vi "Register Discovered Object Instance (incoming).vi"(10 "discoverObjInstance":T1, 11 "hlaMap in":T2) -> (3 "hlaMap out":T2)   [LabVIEW 2019, in "HLA Custom Device Engine.lvlib"]
uses:
  HLA Custom Device Engine.lvlib
  map_object_instance_value.ctl
  _Debug/VsDebugLibrary.lvlib
  map_attr_param_data.ctl
  map_interaction_value.ctl
  map_interaction.ctl
  map_object_value.ctl
  map_object_key.ctl
  map_object.ctl
  map_object_instance.ctl
  map_object_vs_instance.ctl
  RThlaMapHelpers.ctl
  discoverObjectInstance_type.ctl
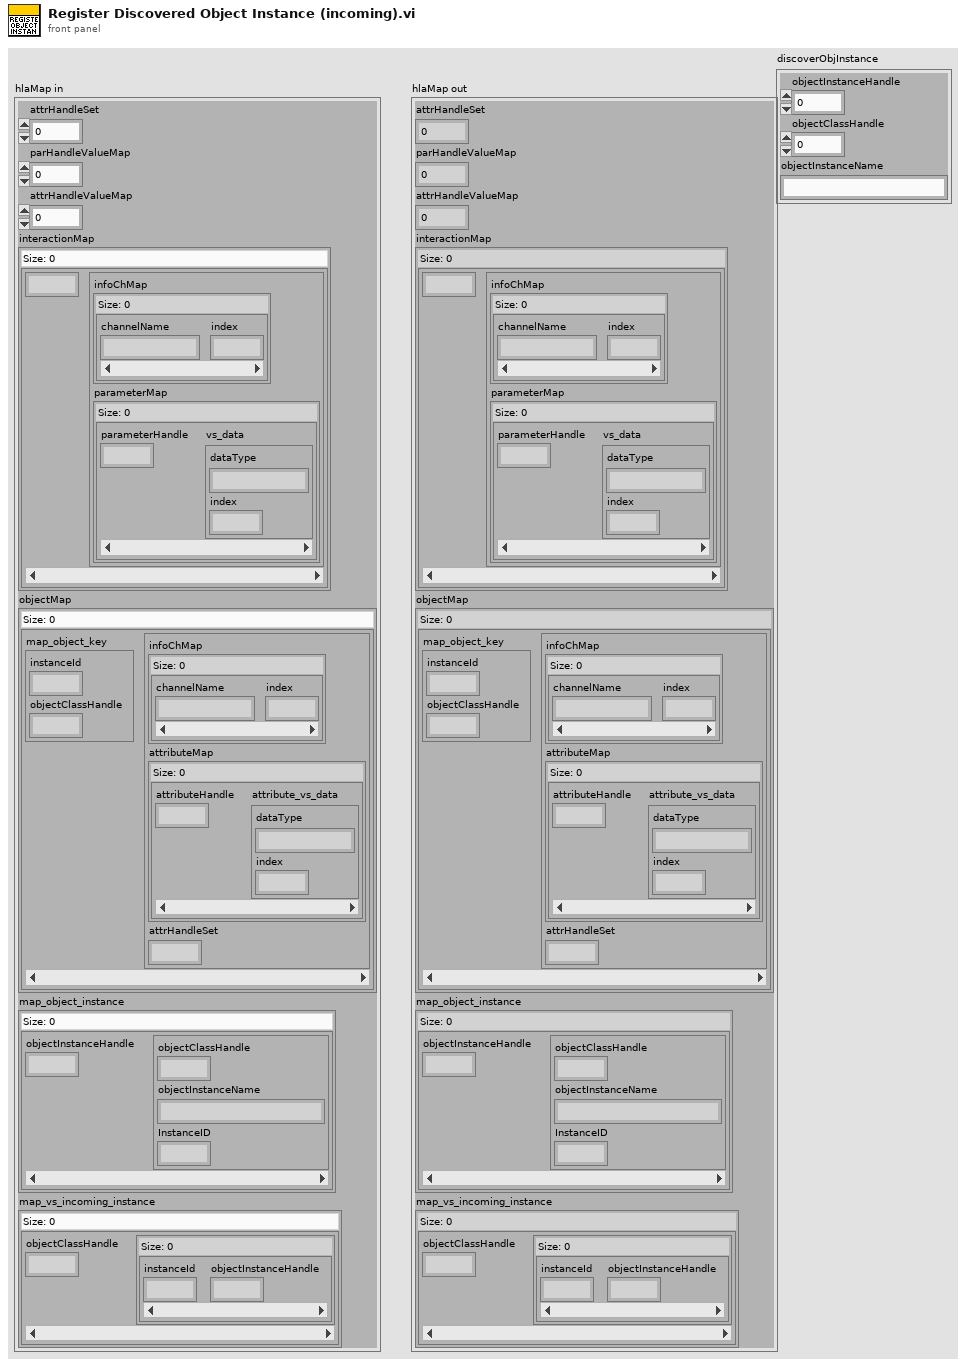
[diagram p1: front panel]
types:
  T1 = typedef "HLA Custom Device Engine.lvlib/discoverObjectInstance_type.ctl" = cluster{"objectInstanceHandle":u64, "objectClassHandle":u64, "objectInstanceName":string}
  T2 = typedef "RThlaMapHelpers.ctl" = cluster{"attrHandleSet":u64, "parHandleValueMap":u64, "attrHandleValueMap":u64, "interactionMap":T3, "objectMap":T6, "map_object_instance":T9, "map_vs_incoming_instance":T11}
  T3 = typedef "HLA Custom Device Engine.lvlib/map_interaction.ctl" = map{u64, T4}
  T4 = typedef "HLA Custom Device Engine.lvlib/map_interaction_value.ctl" = cluster{"infoChMap":map{string, i32}, "parameterMap":map{u64, T5}}
  T5 = typedef "HLA Custom Device Engine.lvlib/map_attr_param_data.ctl" = cluster{"dataType":string, "index":i32}
  T6 = typedef "HLA Custom Device Engine.lvlib/map_object.ctl" = map{T7, T8}
  T7 = typedef "HLA Custom Device Engine.lvlib/map_object_key.ctl" = cluster{"instanceId":i32, "objectClassHandle":u64}
  T8 = typedef "HLA Custom Device Engine.lvlib/map_object_value.ctl" = cluster{"infoChMap":map{string, i32}, "attributeMap":map{u64, T5}, "attrHandleSet":u64}
  T9 = typedef "HLA Custom Device Engine.lvlib/map_object_instance.ctl" = map{u64, T10}
  T10 = typedef "HLA Custom Device Engine.lvlib/map_object_instance_value.ctl" = cluster{"objectClassHandle":u64, "objectInstanceName":string, "InstanceID":i32}
  T11 = typedef "map_object_vs_instance.ctl" = map{u64, map{i32, u64}}
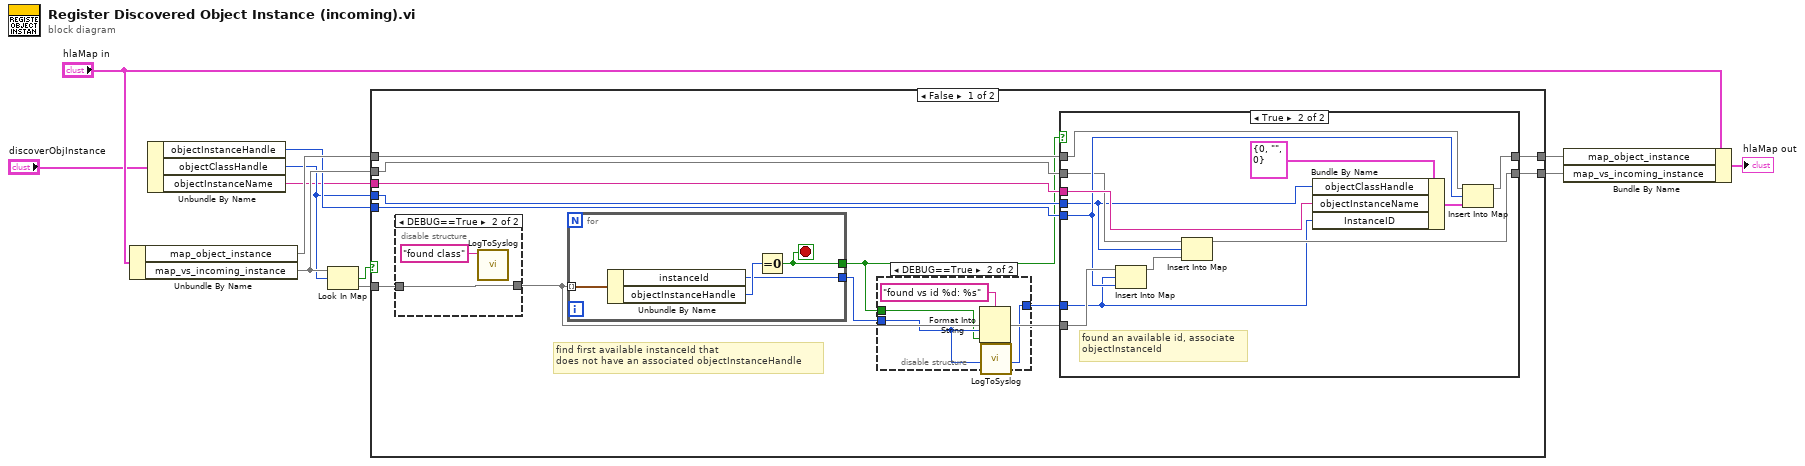
[diagram p0: block diagram]
diagram:
  n1 = Unbundle By Name("hlaMap in") -> ("map_object_instance"=w10:T9, "map_vs_incoming_instance"=w8:T11)
  n2 = Unbundle By Name("discoverObjInstance") -> ("objectInstanceHandle"=w3:u64, "objectClassHandle"=w2:u64, "objectInstanceName"=w1:string)
  n3 = Look In Map(map=w8, key=w2) -> (key not found?=w7:bool, value=w12:map{i32, u64})  [unwired: 1 in]
  n4 = case shown="False" w7 {
    tunnel: w8 -> [w22 w50]
    tunnel: [w18 w50] -> w9
    tunnel: w10 -> [w21 w49]
    tunnel: [w20 w49] -> w11
    tunnel: w12 -> [w16 _]
    tunnel: w3 -> [w19 _]
    tunnel: w2 -> [w24 _]
    tunnel: w1 -> [w23 _]
    frame False {
      # "find first available instanceId that\ndoes not have an associated objectInstanceHandle"
      n5 = disable-structure shown="DEBUG==True" {
        disable-tunnel: [_ w30] -> w17
        disable-tunnel: w16 -> [_ w30]
        frame condition #0 {
        }
        frame condition #1 (active) {
          n6 = call "LogToSyslog.vi"("message"="found class") -> ()  [unwired: 9 in, 2 out]
        }
      }
      n7 = for {
        tunnel: w17 -> [w48] mode=indexing
        tunnel: [w46] -> w13
        tunnel: [w45] -> w15
        stop <- w46 stop-if-true
        n8 = Unbundle By Name(w48) -> ("instanceId"=w45:i32, "objectInstanceHandle"=w47:u64)
        n9 = Equal To 0?(x=w47) -> (x = 0?=w46:bool)
      }
      n10 = disable-structure shown="DEBUG==True" {
        disable-tunnel: w15 -> [_ w26]
        disable-tunnel: [_ w26] -> w14
        disable-tunnel: w13 -> [_ w25]
        frame condition #0 {
        }
        frame condition #1 (active) {
          n11 = Format Into String(format string="found vs id %d: %s" ("message"), w26, w25) -> (resulting string=w27:string)  [unwired: 2 in, 1 out]
          n12 = call "LogToSyslog.vi"("message"=w27) -> ()  [unwired: 9 in, 2 out]
        }
      }
      n13 = case shown="True" w13 {
        tunnel: w24 -> [_ w35]
        tunnel: w23 -> [_ w43]
        tunnel: w17 -> [_ w39]
        tunnel: w22 -> [w31 w37]
        tunnel: w21 -> [w32 w42]
        tunnel: [w32 w41] -> w20
        tunnel: w19 -> [_ w38]
        tunnel: [w31 w34] -> w18
        tunnel: w14 -> [_ w33]
        frame False {
        }
        frame True {
          # "found an available id, associate\nobjectInstanceId"
          n14 = Insert Into Map(map in=w39, key=w33, value=w38) -> (map out=w36:map{i32, u64})  [unwired: 2 out]
          n15 = Insert Into Map(map in=w37, key=w35, value=w36) -> (map out=w34:T11)  [unwired: 2 out]
          n16 = Bundle By Name(cluster=T10 {"objectClassHandle"=0, "objectInstanceName"="", "InstanceID"=0} ("value"), "objectClassHandle"=w35, "objectInstanceName"=w43, "InstanceID"=w33) -> (w40:T10)
          n17 = Insert Into Map(map in=w42, key=w38, value=w40) -> (map out=w41:T9)  [unwired: 2 out]
        }
      }
    }
    frame True {
    }
  }
  n18 = Bundle By Name(cluster="hlaMap in", "map_object_instance"=w11, "map_vs_incoming_instance"=w9) -> (→"hlaMap out":T2)
